vi "GetXML.vi"(0 "Node ROS":T2={"topic port"=0, "Node"="", "topic"="", "type"="", "node port"=0, "error "={"status"=FALSE, "code"=0, "source"=""}, "Direction"=enum."Node", "APIs"=[], "Update (ms)"=1, "write queue"=1}, 1 "Subscribers in":T1(array[cluster])) -> (3 "reply":string, 4 "Subscribers Out":T1(array[cluster]))   [LabVIEW 2012]
uses:
  <userlib>/ROSforLV/ROS/Code/SubVIs/_ROSControl.ctl
  <userlib>/ROSforLV/ROS/Code/SubVIs/_ROSDirection.ctl
  <userlib>/ROSforLV/ROS/Code/Console/Servers/ServerSubs/ROSLog.ctl
  <userlib>/ROSforLV/ROS/Code/_ROSDefinition.vi
  <userlib>/ROSforLV/ROS/MessageBuilding/std_msgs/subs/i16Scalar.vi
  <userlib>/ROSforLV/ROS/MessageBuilding/std_msgs/subs/stringScalar.vi
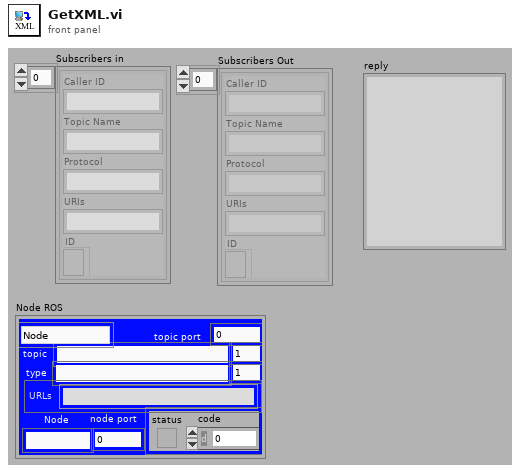
[diagram p1: front panel]
types:
  T1 = cluster{"Caller ID":string, "Topic Name":string, "Protocol":string, "URIs":string, "ID":refnum<k5>}[]
  T2 = typedef "_ROSControl.ctl" = cluster{"topic port":u16, "Node":string, "topic":string, "type":string, "node port":u32, "error ":errorcluster, "Direction":T3, "APIs":string[], "Update (ms)":u16, "write queue":u16}
  T3 = typedef "_ROSDirection.ctl" = enum16{"Node", "Publisher", "Subscriber", "Service Client"}
  T4 = typedef "ROSLog.ctl" = cluster{"Sent":string, "Reply":string, "MethodName":string, "success":bool, "Dir1":string, "Dir2":string, "Time Stamp":string, "error":errorcluster, "Preamble":string}
  T5 = enum16{"Add Server", "Clear Server", "Clear All", "Get Info", "GetPanelInfo"}
  T6 = cluster{"Caller ID":string, "Topic Name":string, "Protocol":string, "URIs":string, "ID":refnum<k5>}
  T7 = typedef "requestTopic.ctl" = cluster{"New Subscriber":cluster{"Caller ID":string, "Topic Name":string, "Protocol":string, "URIs":string, "ID":refnum<k5>}, "ROS of Server":T2, "new port":u16}
  T8 = typedef "MyState.ctl" = enum16{"No Connection", "Registered", "Connected", "Close"}
  T9 = typedef "ServoInfo.ctl" = cluster{"vi name":string, "VI Refnum":refnum<vi>, "queue":refnum<queue>, "ROS":T2, "notifier":refnum<notifier>}
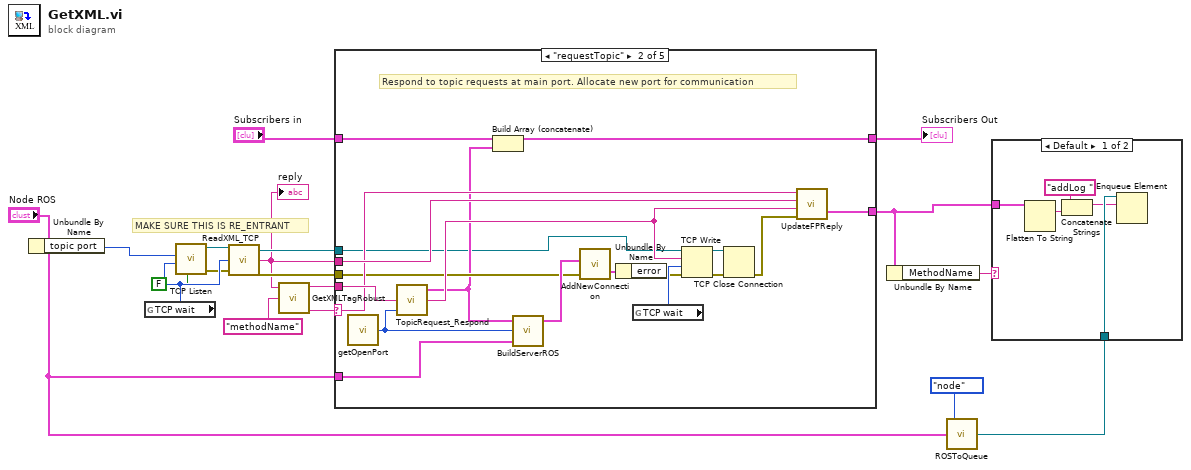
[diagram p0: block diagram]
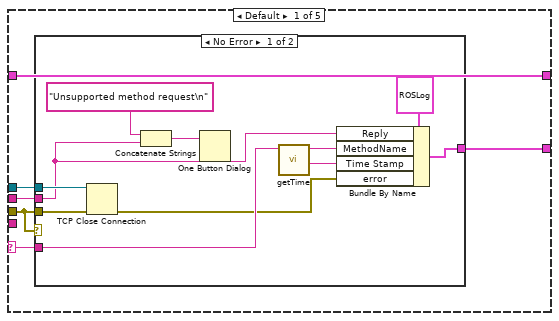
[diagram p3: hidden frame]
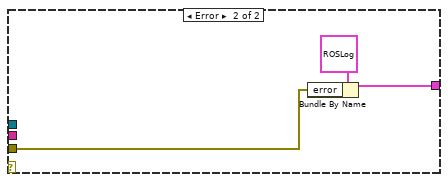
[diagram p4: hidden frame]
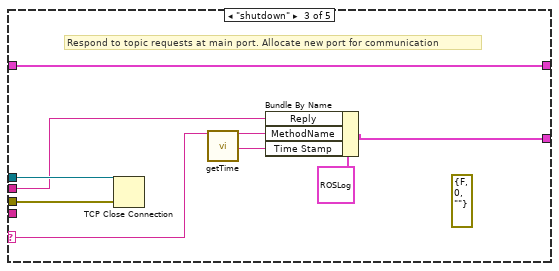
[diagram p5: hidden frame]
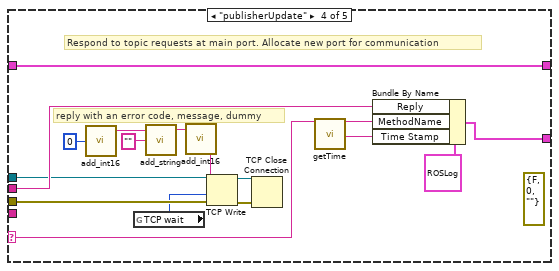
[diagram p6: hidden frame]
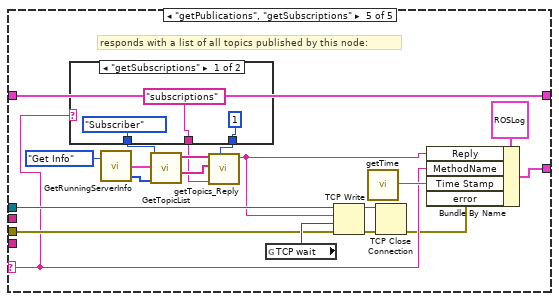
[diagram p7: hidden frame]
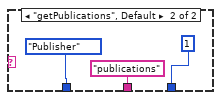
[diagram p8: hidden frame]
diagram:
  # "MAKE SURE THIS IS RE_ENTRANT"
  n1 = Unbundle By Name("Node ROS") -> ("topic port"=w7:u16)
  n2 = global read "_ROSDefinition.vi" "TCP wait"() -> (w5:i32)
  n3 = call <vilib>:"TCP Listen.vi"("resolve remote address (T)"=FALSE, "timeout ms (wait forever: -1)"=w5, "port"=w7) -> ("error out"=w4:errorcluster, "connection ID"=w6:refnum<k5>)  [unwired: 4 in, 3 out]
  n4 = call <userlib>:"ReadXML_TCP.vi"("error in"=w4, "timeout ms (3000)"=w5, "connection ID in"=w6) -> ("error out"=w17:errorcluster, "data out"=w9:string, "connection ID out"=w16:refnum<k5>)
  "reply" <- w9
  n5 = call <userlib>:"GetXMLTagRobust.vi"("Tag"="methodName", "String"=w9) -> ("value"=w13:string, "String w/o Tag"=w14:string)  [unwired: 1 in, 2 out]
  n6 = case shown="\"requestTopic\"" w13 {
    selector: w13 -> [w22 w53 w59 w77 w86]
    tunnel: w14 -> [_ w56 _ _ _]
    tunnel: "Subscribers in" -> [w24 w48 w64 w80 w100]
    tunnel: w16 -> [w23 w41 w63 w69 w93]
    tunnel: w17 -> [w20 w49 w62 w70 w92]
    tunnel: [w24 w47 w64 w80 w100] -> w18
    tunnel: "Node ROS" -> [_ w44 _ _ _]
    tunnel: w9 -> [w21 w54 w60 w78 _]
    tunnel: [w19 w46 w57 w75 w99] -> w2
    frame Default {
      n7 = case shown="No Error" w20 {
        tunnel: w23 -> [w34 _]
        tunnel: w20 -> [w33 w36]
        tunnel: [w28 w35] -> w19
        tunnel: w22 -> [w27 _]
        tunnel: w21 -> [w26 _]
        frame No Error {
          n8 = TCP Close Connection(connection ID=w34, error in (no error)=w33) -> (error out=w25:errorcluster)  [unwired: 1 in, 1 out]
          n9 = Concatenate Strings("Unsupported method request\n" ("message"), w26) -> (w31:string)
          n10 = One Button Dialog(message=w31) -> ()  [unwired: 1 in, 1 out]
          n11 = call <userlib>:"getTime.vi"() -> ("Current Time"=w29:string)  [unwired: 1 in]
          n12 = Bundle By Name(cluster=T4 {"Sent"="", "Reply"="", "MethodName"="", "success"=FALSE, "Dir1"="To ROS", "Dir2"="From ROS", "Time Stamp"="", "error"={"status"=FALSE, "code"=0, "source"=""}, "Preamble"=""} ("Log"), "Reply"=w26, "MethodName"=w27, "Time Stamp"=w29, "error"=w25) -> (w28:T4)
        }
        frame Error {
          n13 = Bundle By Name(cluster=T4 {"Sent"="TCP Read Error in Node", "Reply"="", "MethodName"="Node read error", "success"=FALSE, "Dir1"="To ROS", "Dir2"="From ROS", "Time Stamp"="", "error"={"status"=FALSE, "code"=0, "source"=""}, "Preamble"=""} ("Log"), "error"=w36) -> (w35:T4)
        }
      }
    }
    frame "requestTopic" {
      # "Respond to topic requests at main port. Allocate new port for communication"
      n14 = call <userlib>:"getOpenPort.vi"() -> ("port"=w43:u16)
      n15 = call <userlib>:"TopicRequest_Respond.vi"("port"=w43, "XML"=w56) -> ("Topic Request Reply"=w52:string, "New Subscriber"=w42:T6)  [unwired: 2 in]
      n16 = Build Array (concatenate)(w48, w42) -> (w47:T1)
      n17 = call <userlib>:"BuildServerROS.vi"("Node ROS"=w44, "port"=w43, "New Subscriber"=w42) -> ("data"=w50:T7)  [unwired: 2 in]
      n18 = call <userlib>:"AddNewConnection.vi"("error in (no error)"=w49, "data"=w50) -> ("Log"=w39:T4)  [unwired: 3 in]
      n19 = Unbundle By Name(w39) -> ("error"=w38:errorcluster)
      n20 = global read "_ROSDefinition.vi" "TCP wait"() -> (w45:i32)
      n21 = TCP Write(connection ID=w41, data in=w52, error in (no error)=w38, 9:w45) -> (connection ID out=w55:refnum<k5>, error out=w51:errorcluster)  [unwired: 1 out]
      n22 = TCP Close Connection(connection ID=w55, error in (no error)=w51) -> (error out=w40:errorcluster)  [unwired: 1 in, 1 out]
      n23 = call <userlib>:"UpdateFPReply.vi"("error in (no error)"=w40, "Reply"=w52, "Sent"=w54, "method"=w53) -> ("Log"=w46:T4)
    }
    frame "shutdown" {
      (unwired) errorcluster {"status"=FALSE, "code"=0, "source"=""} ("error IO")
      # "Respond to topic requests at main port. Allocate new port for communication"
      n24 = TCP Close Connection(connection ID=w63, error in (no error)=w62) -> ()  [unwired: 1 in, 2 out]
      n25 = call <userlib>:"getTime.vi"() -> ("Current Time"=w58:string)  [unwired: 1 in]
      n26 = Bundle By Name(cluster=T4 {"Sent"="", "Reply"="", "MethodName"="", "success"=FALSE, "Dir1"="To ROS", "Dir2"="From ROS", "Time Stamp"="", "error"={"status"=FALSE, "code"=0, "source"=""}, "Preamble"=""} ("Log"), "Reply"=w60, "MethodName"=w59, "Time Stamp"=w58) -> (w57:T4)
    }
    frame "publisherUpdate" {
      (unwired) errorcluster {"status"=FALSE, "code"=0, "source"=""} ("error IO")
      # "reply with an error code, message, dummy"
      # "Respond to topic requests at main port. Allocate new port for communication"
      n27 = call-poly <userlib>:"add_int16.vi"("Numeric"=i16 0) -> ("msg out"=w74:string)  [unwired: 4 in]
      n28 = global read "_ROSDefinition.vi" "TCP wait"() -> (w68:i32)
      n29 = call-poly <userlib>:"add_string.vi"("String"="", "msg in"=w74) -> ("msg out"=w73:string)  [unwired: 3 in]
      n30 = call-poly <userlib>:"add_int16.vi"("msg in"=w73) -> ("msg out"=w67:string)  [unwired: 4 in]
      n31 = TCP Write(connection ID=w69, data in=w67, error in (no error)=w70, 9:w68) -> (connection ID out=w66:refnum<k5>, error out=w65:errorcluster)  [unwired: 1 out]
      n32 = TCP Close Connection(connection ID=w66, error in (no error)=w65) -> ()  [unwired: 1 in, 2 out]
      n33 = call <userlib>:"getTime.vi"() -> ("Current Time"=w76:string)  [unwired: 1 in]
      n34 = Bundle By Name(cluster=T4 {"Sent"="", "Reply"="", "MethodName"="", "success"=FALSE, "Dir1"="To ROS", "Dir2"="From ROS", "Time Stamp"="", "error"={"status"=FALSE, "code"=0, "source"=""}, "Preamble"=""} ("Log"), "Reply"=w78, "MethodName"=w77, "Time Stamp"=w76) -> (w75:T4)
    }
    frame "getPublications", "getSubscriptions" {
      # "responds with a list of all topics published by this node:"
      n35 = case shown="\"getSubscriptions\"" w86 {
        tunnel: [_ROSDirection."Subscriber" ("ROS.Direction") _ROSDirection."Publisher" ("ROS.Direction")] -> w85
        tunnel: [1 ("Code") 1 ("Code")] -> w83
        tunnel: ["subscriptions" ("StatusMessage") "publications" ("StatusMessage")] -> w82
        frame "getSubscriptions" {
        }
        frame "getPublications", Default {
        }
      }
      n36 = call <userlib>:"GetRunningServerInfo.vi"("Task"=T5."Get Info") -> ("Status"=w89:T8[], "servers"=w90:T9[])  [unwired: 1 in, 1 out]
      n37 = call <userlib>:"GetTopicList.vi"("Status"=w89, "servers"=w90, "ROS.Direction"=w85) -> ("Topic Types"=w84:string[], "Topics"=w88:string[])  [unwired: 7 in]
      n38 = call <userlib>:"getTopics_Reply.vi"("Code"=w83, "StatusMessage"=w82, "Topic Types"=w84, "Topics"=w88) -> ("XML Out"=w87:string)  [unwired: 7 in]
      n39 = global read "_ROSDefinition.vi" "TCP wait"() -> (w96:i32)
      n40 = TCP Write(connection ID=w93, data in=w87, error in (no error)=w92, 9:w96) -> (connection ID out=w94:refnum<k5>, error out=w95:errorcluster)  [unwired: 1 out]
      n41 = call <userlib>:"getTime.vi"() -> ("Current Time"=w97:string)  [unwired: 1 in]
      n42 = TCP Close Connection(connection ID=w94, error in (no error)=w95) -> (error out=w81:errorcluster)  [unwired: 1 in, 1 out]
      n43 = Bundle By Name(cluster=T4 {"Sent"="", "Reply"="", "MethodName"="", "success"=FALSE, "Dir1"="To ROS", "Dir2"="From ROS", "Time Stamp"="", "error"={"status"=FALSE, "code"=0, "source"=""}, "Preamble"=""} ("Log"), "Reply"=w87, "MethodName"=w86, "Time Stamp"=w97, "error"=w81) -> (w99:T4)
    }
  }
  "Subscribers Out" <- w18
  n44 = Unbundle By Name(w2) -> ("MethodName"=w1:string)
  n45 = call <userlib>:"ROSToQueue.vi"("ROS"="Node ROS", "Name"=enum16{"topic", "node"}."node") -> ("queue"=w10:refnum<queue>)  [unwired: 2 in, 1 out]
  n46 = case shown="Default" w1 {
    tunnel: w10 -> [w111 _]
    tunnel: w2 -> [w110 _]
    frame Default {
      n47 = Flatten To String(anything=w110) -> (data string=w108:string)  [unwired: 3 in, 2 out]
      n48 = Concatenate Strings("addLog " ("string"), w108) -> (w109:string)
      n49 = Enqueue Element(queue=w111, element=w109) -> ()  [unwired: 2 in, 3 out]
    }
    frame "" {
    }
  }
